vi "Check Divisable.vi"() -> ()   [LabVIEW 2020]
uses:
  2130b342-8d85-4ad8-a0a8-91cc1bda410b.vi
  <vilib>/Comparison/Less/Less Functor/Less Functor.lvclass
panel:
  out "multiple remainder":u64
  out "divisable":bool
  in  "divisor":u64
  in  "Add":u64
  in  "multiplyers":u64[](array[numeric])
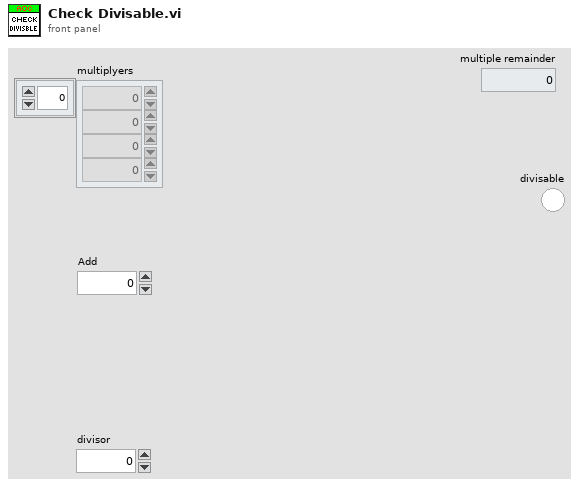
[diagram p1: front panel]
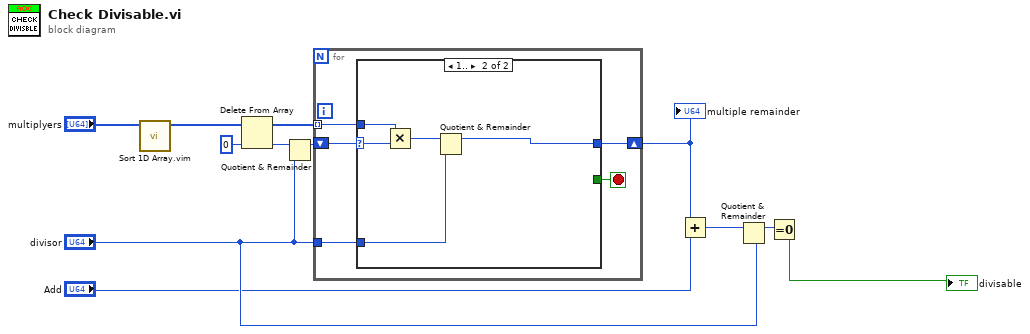
[diagram p0: block diagram]
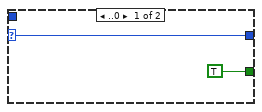
[diagram p2: hidden frame]
diagram:
  n1 = call "Sort 1D Array.vim"("unsorted array"="multiplyers") -> ("sorted array"=w6:u64[])  [unwired: 10 in]
  n2 = Delete From Array(array=w6, index=0) -> (deleted portion=w5:u64, array with subset deleted=w3:u64[])  [unwired: 1 in]
  n3 = Quotient & Remainder(x=w5, y="divisor") -> (x-y*floor(x/y)=w4:u64)  [unwired: 1 out]
  n4 = for {
    tunnel: "divisor" -> [w15]
    shift-right: [w14] -> w1
    shift-left: w4 -> [w16]
    tunnel: w3 -> [w17] mode=indexing
    stop <- w13 stop-if-true
    n5 = case shown="1.." w16 {
      selector: w16 -> [w19 w23]
      tunnel: w17 -> [_ w24]
      tunnel: w15 -> [_ w21]
      tunnel: [w19 w20] -> w14
      tunnel: [TRUE _] -> w13
      frame ..0 {
      }
      frame 1.. {
        n6 = Multiply(x=w24, y=w23) -> (x*y=w22:u64)
        n7 = Quotient & Remainder(x=w22, y=w21) -> (x-y*floor(x/y)=w20:u64)  [unwired: 1 out]
      }
    }
  }
  "multiple remainder" <- w1
  n8 = Add(x=w1, y="Add") -> (x+y=w8:u64)
  n9 = Quotient & Remainder(x=w8, y="divisor") -> (x-y*floor(x/y)=w7:u64)  [unwired: 1 out]
  n10 = Equal To 0?(x=w7) -> (x = 0?=→"divisable":bool)
